vi "svx_Check Channel Property and Pair.vi"(7 "reset in":bool, 8 "error in (no error)":errorcluster, 10 "channel number":i32, 11 "channel property":T1[](array[typedef]) {"probe angle [deg]" max=360; "direction" items=["CCW", "CW"]}) -> (0 "error out":errorcluster, 3 "channel property out":T1[](array[typedef]) {"probe angle [deg]" max=360; "direction" items=["CCW", "CW"]}, 5 "reset out":bool)   [LabVIEW 2017]
uses:
  <vilib>/addons/Sound and Vibration/Order Analysis/Data Presentation/SubVIs/OAT MCM Channel Property.ctl
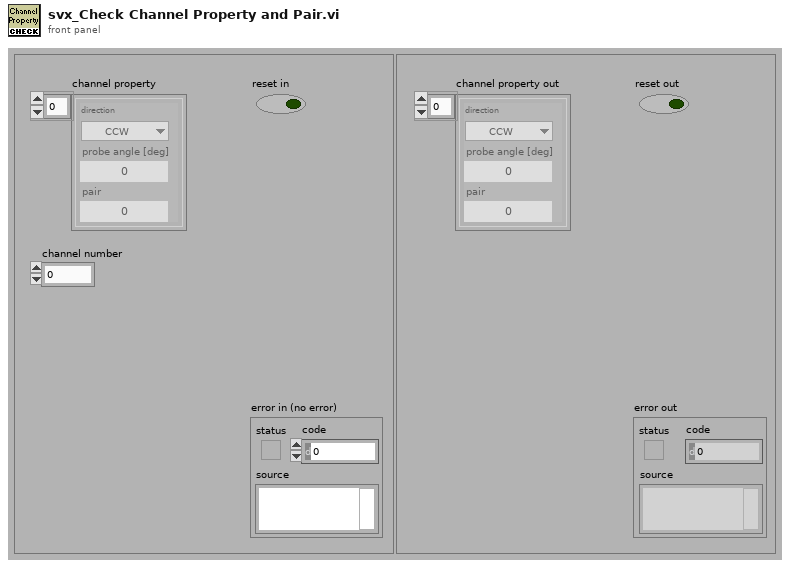
[diagram p1: front panel]
types:
  T1 = typedef "OAT MCM Channel Property.ctl" = cluster{"direction":u16, "probe angle [deg]":u16, "pair":u16}
  T2 = cluster{"direction":u16, "probe angle [deg]":u16, "pair":u16}
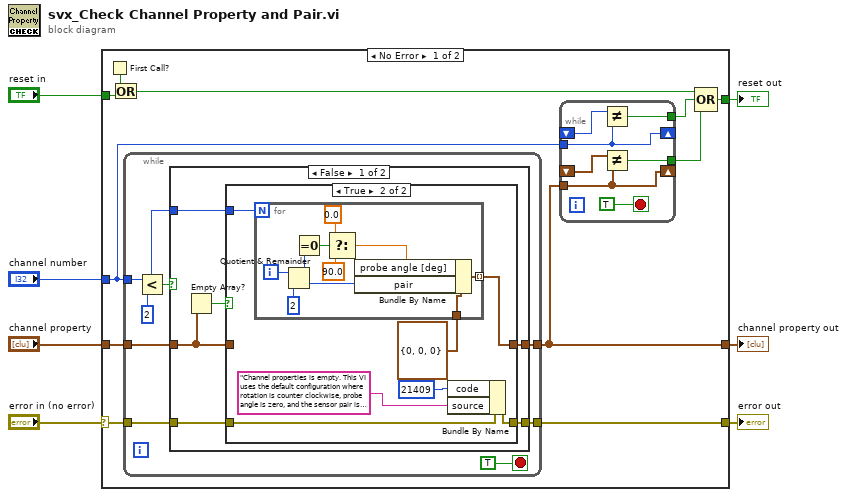
[diagram p0: block diagram]
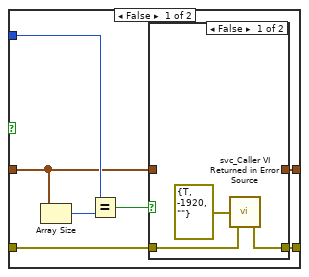
[diagram p2: hidden frame]
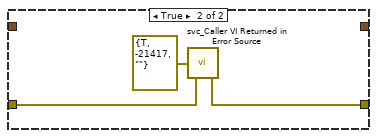
[diagram p4: hidden frame]
diagram:
  n1 = case shown="No Error" "error in (no error)" {
    selector: "error in (no error)" -> [w18 w72]
    tunnel: [w17 w72] -> w6
    tunnel: "channel property" -> [w16 w73]
    tunnel: [w8 w73] -> w4
    tunnel: "channel number" -> [w13 _]
    tunnel: "reset in" -> [w15 _]
    tunnel: [w9 _] -> w1
    frame No Error {
      n2 = First Call?() -> (First Call?: T/F=w14:bool)
      n3 = Or(x=w14, y=w15) -> (x .or. y?=w10:bool)
      n4 = while {
        tunnel: w18 -> [w33]
        tunnel: [w32] -> w17
        tunnel: [w29] -> w8
        tunnel: w16 -> [w28]
        tunnel: w13 -> [w26]
        stop <- TRUE stop-if-true
        n5 = Less?(x=w26, y=2) -> (x < y?=w27:bool)
        n6 = case shown="False" w27 {
          tunnel: w33 -> [w38 w70]
          tunnel: [w37 w69] -> w32
          tunnel: w26 -> [w35 _]
          tunnel: w28 -> [w39 _]
          tunnel: [w36 _] -> w29
          frame False {
            n7 = Empty Array?(array=w39) -> (empty?=w34:bool)
            n8 = case shown="True" w34 {
              tunnel: w39 -> [w44 _]
              tunnel: w35 -> [w45 w58]
              tunnel: w38 -> [w42 w57]
              tunnel: [w41 w56] -> w37
              tunnel: [w43 w54] -> w36
              frame False {
                n9 = Array Size(array=w44) -> (size(s)=w46:i32)
                n10 = Equal?(x=w45, y=w46) -> (x = y?=w40:bool)
                n11 = case shown="False" w40 {
                  tunnel: w44 -> [_ w51]
                  tunnel: [_ w51] -> w43
                  tunnel: w42 -> [w48 w50]
                  tunnel: [w47 w50] -> w41
                  frame False {
                    n12 = call <vilib>:"svc_Caller VI Returned in Error Source.vi"("warning input to caller"=w48, "error in (no error)"=errorcluster {"status"=TRUE, "code"=-1920, "source"=""} ("error out")) -> ("error out"=w47:errorcluster)  [unwired: 3 in]
                  }
                  frame True {
                  }
                }
              }
              frame True {
                n13 = for {
                  N: w58 -> [_]
                  tunnel: [w60] -> w54 mode=indexing
                  tunnel: T2 {"direction"=0, "probe angle [deg]"=0, "pair"=0} ("channel property") -> [w59]
                  i -> [w68]
                  n14 = Quotient & Remainder(x=w68, y=2) -> (x-y*floor(x/y)=w65:i32, floor(x/y)=w66:i32)
                  n15 = Equal To 0?(x=w65) -> (x = 0?=w64:bool)
                  n16 = Select(t=0.0 ("probe angle [deg]"), s=w64, f=90.0) -> (s? t:f=w61:dbl)
                  n17 = Bundle By Name(cluster=w59, "probe angle [deg]"=w61, "pair"=w66) -> (w60:T2)
                }
                n18 = Bundle By Name(cluster=w57, "code"=21409, "source"="Channel properties is empty. This VI uses the default configuration where rotation is counter clockwise, probe angle is zero, and the sensor pair is determined by the channel index.") -> (w56:errorcluster)
              }
            }
          }
          frame True {
            n19 = call <vilib>:"svc_Caller VI Returned in Error Source.vi"("warning input to caller"=w70, "error in (no error)"=errorcluster {"status"=TRUE, "code"=-21417, "source"=""} ("error out")) -> ("error out"=w69:errorcluster)  [unwired: 3 in]
          }
        }
      }
      n20 = while {
        tunnel: w8 -> [w23]
        tunnel: w13 -> [w24]
        shift-right: [w24] -> _
        shift-left: _ -> [w25]
        shift-right: [w23] -> _
        shift-left: _ -> [w22]
        tunnel: [w20] -> w12
        tunnel: [w19] -> w11
        stop <- TRUE stop-if-true
        n21 = Not Equal?(x=w25, y=w24) -> (x != y?=w19:bool)
        n22 = Not Equal?(x=w22, y=w23) -> (x != y?=w20:bool)
      }
      n23 = Compound Arithmetic op=OR(w10, w11, w12) -> (w9:bool)
    }
    frame Error {
    }
  }
  "error out" <- w6
  "channel property out" <- w4
  "reset out" <- w1
